vi "X sort to color-20220125.vi"(6 "Array 6":dbl[](array[numeric]), 9 "Array 4":dbl[][](array[numeric]), 10 "Array 5":dbl[][](array[numeric]), 11 "Array in":u32[](array[numeric])) -> (2 "Array 3":dbl[](array[numeric]), 3 "Array out":u32[](array[numeric]))   [LabVIEW 2019]
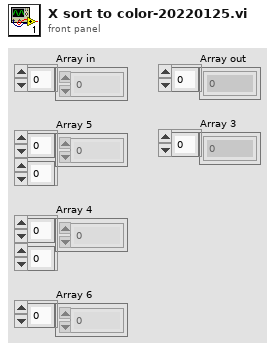
[diagram p1: front panel]
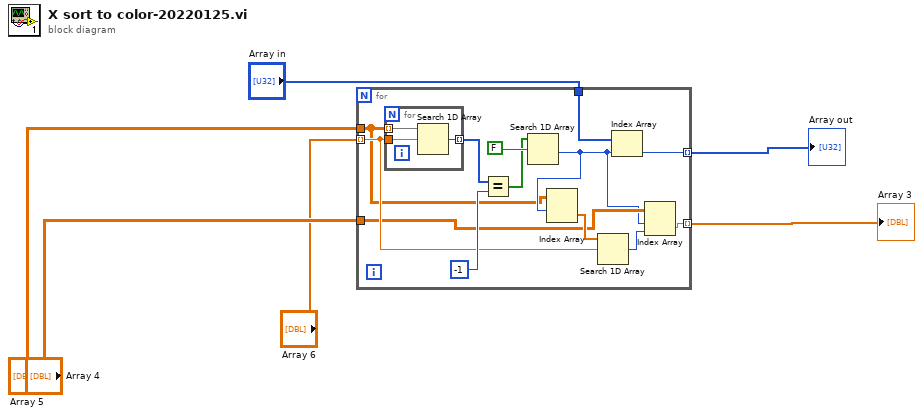
[diagram p0: block diagram]
diagram:
  n1 = for {
    tunnel: "Array 6" -> [w13] mode=indexing
    tunnel: "Array 5" -> [w7]
    tunnel: "Array in" -> [w16]
    tunnel: [w15] -> w6 mode=indexing
    tunnel: "Array 4" -> [w10]
    tunnel: [w11] -> w4 mode=indexing
    n2 = for {
      tunnel: w7 -> [w22] mode=indexing
      tunnel: w13 -> [w21]
      tunnel: [w20] -> w19 mode=indexing
      n3 = Search 1D Array(1D array=w22, element=w21) -> (index of element=w20:i32)  [unwired: 1 in]
    }
    n4 = Equal?(x=w19, y=-1) -> (x = y?=w14:bool[])
    n5 = Search 1D Array(1D array=w14, element=FALSE) -> (index of element=w8:i32)  [unwired: 1 in]
    n6 = Index Array(array=w7, index (row)=w8) -> (element=w12:dbl[])  [unwired: 1 in]
    n7 = Search 1D Array(1D array=w12, element=w13) -> (index of element=w9:i32)  [unwired: 1 in]
    n8 = Index Array(array=w16, index=w8) -> (element=w15:u32)
    n9 = Index Array(array=w10, index (row)=w8, index (col)=w9) -> (element=w11:dbl)
  }
  "Array out" <- w6
  "Array 3" <- w4
